vi "_Remote Set CEM.vi"(4 "error in":errorcluster, 6 "CEM (0V)":dbl, 7 "Use Default (F)":bool) -> (0 "error out":errorcluster)   [LabVIEW 2012]
uses:
  Type/_RT Command.ctl
  Type/_RT Parameter.ctl
  Type/_RT Active Ch.ctl
  Type/_RT Expt.ctl
  Type/_Run Mode.ctl
  Type/_RT Mass Range.ctl
  Type/_RT Res Type.ctl
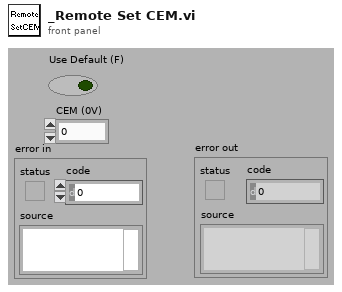
[diagram p1: front panel]
types:
  T1 = typedef "_RT Configuration 2.ctl" = cluster{"Name":string, "Ch#":u8, "Min":dbl, "Max":dbl, "Def+":dbl, "Def-":dbl, "Offset":dbl, "Slope":dbl, "Type":u8, "Description":string, "SettleT":dbl}
  T2 = typedef "_RT Active Ch.ctl" = cluster{"Start":i32, "Step":i32, "ChID":i32}
  T3 = typedef "_RT Command.ctl" = enum16{"Start", "Stop", "Runtime Update", "Get Data", "Get Info", "Get Status", "Get Param", "Get Config", "Get Table", "Read ADC", "Set Oscillator", "Update Config", "Update Table", "Set All Pol", "Set Pol and DC", "Set Max Mass", "Toggle RP", "Toggle EL", "Set PIC", "Initialize Turbo", "Send Turbo Comm", "Close Turbo", "P1", "P2", "P3", "Send Serial", "Set LC Out", "Get LC In", "Read VAC", "Test Table", "Toggle Power", "Get Startup", "Set Startup", "Get ADC Table", "Set ADC Table", "Get Brief Status", "Get Detail Status", "Auxiliary Update", "Set CC Logics", "Set CC Input Logics", "Ignore Error"}
  T4 = typedef "_RT Expt.ctl" = cluster{"StartT(mS)":i32, "#Cycles":i32, "Scan Type":T5, "PauseT(uS)":i32, "Polarity":u8, "DelayT(mS)":i32, "Active Ch":T2[], "Mass Range":T6[]}
  T5 = typedef "_Run Mode.ctl" = enum16{"MRM (Q1/Q2)", "Q1 Scan", "Q1 SRM", "Q2 Scan", "Q2 SRM", "Product Scan", "Precursor Scan", "Neutral Loss", "Neutral Gain"}
  T6 = typedef "_RT Mass Range.ctl" = cluster{"Steps":i32, "Dwell(uS)":i32, "Resolution Type":T7, "Ramping Ch":T2[]}
  T7 = typedef "_RT Res Type.ctl" = u16
  T8 = typedef "_RT Parameter.ctl" = cluster{"RunMode":i32, "Initial Ch":T2[], "Sync":u8, "Expt":T4[], "EqTime(mS)":i32}
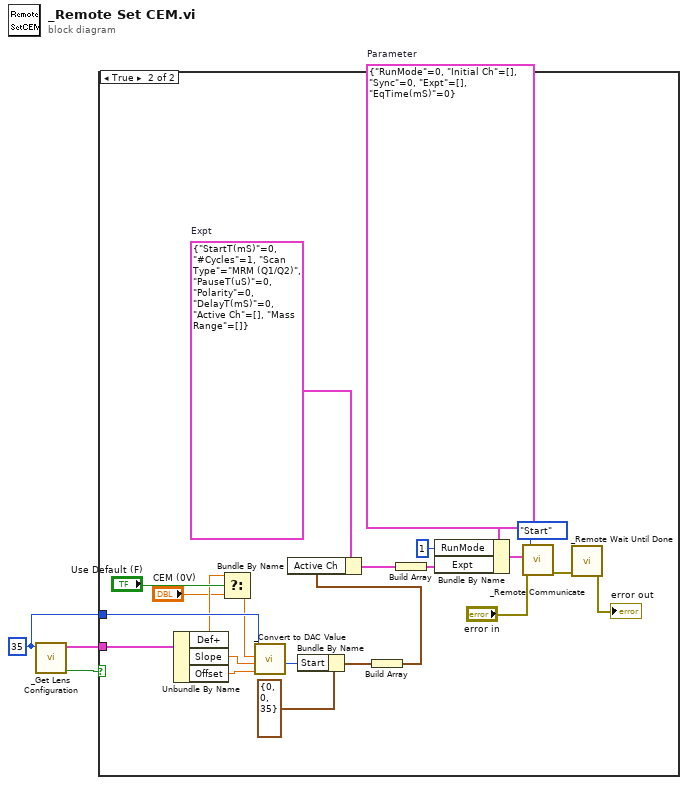
[diagram p0: block diagram]
diagram:
  w2 = u8 35 ("Channel #")
  n1 = call "_Get Lens Configuration.vi"("Channel #"=w2) -> ("Found"=w1:bool, "Lens Configuration"=w3:T1)  [unwired: 1 in, 4 out]
  n2 = case shown="True" w1 {
    tunnel: w3 -> [_ w9]
    tunnel: w2 -> [_ w8]
    frame False {
    }
    frame True {
      w19 = T4 {"StartT(mS)"=0, "#Cycles"=1, "Scan Type"=enum."MRM (Q1/Q2)", "PauseT(uS)"=0, "Polarity"=0, "DelayT(mS)"=0, "Active Ch"=[], "Mass Range"=[]}  # Expt
      w22 = T8 {"RunMode"=0, "Initial Ch"=[], "Sync"=0, "Expt"=[], "EqTime(mS)"=0}  # Parameter
      n3 = Unbundle By Name(w9) -> ("Def+"=w6:dbl, "Slope"=w12:dbl, "Offset"=w11:dbl)
      n4 = Select(t=w6, s="Use Default (F)", f="CEM (0V)") -> (s? t:f=w5:dbl)
      n5 = call "_Convert to DAC Value.vi"("Offset"=w11, "Slop"=w12, "Number"=w5, "Channel"=w8) -> ("DAC Value"=w10:i32)  [unwired: 2 in, 5 out]
      n6 = Bundle By Name(cluster=T2 {"Start"=0, "Step"=0, "ChID"=35} ("output cluster"), "Start"=w10) -> (w14:T2)
      n7 = Build Array(w14) -> (w13:T2[])
      n8 = Bundle By Name(cluster=w19, "Active Ch"=w13) -> (w18:T4)
      n9 = Build Array(w18) -> (w17:T4[])
      n10 = Bundle By Name(cluster=w22, "RunMode"=1, "Expt"=w17) -> (w21:T8)
      n11 = call "_Remote Communicate.vi"("error in (no error)"="error in", "Parameter"=w21, "Command"=_RT_Command."Start") -> ("error out"=w23:errorcluster)  [unwired: 3 in, 3 out]
      n12 = call "_Remote Wait Until Done.vi"("error IO"=w23) -> ("error out"=→"error out":errorcluster)  [unwired: 1 in, 1 out]
    }
  }
